vi "GitHub OAuth Test.vi"() -> ()   [LabVIEW 2013]
uses:
  source/OauthClient/OAuthClient.lvclass
  source/Oauth2/Oauth2.lvclass/Oauth2.ctl
  source/Oauth2/Oauth2.lvclass
  source/Oauth2.Github/Oauth2.GitHub.lvclass
  <vilib>/LabVIEW Open Source Project/OpenURI/uri/URI.lvclass
  <vilib>/httpClient/LabVIEWHTTPClient.lvlib
panel:
  out "GitHub Root":string
  out "HTTP Response Headers":string
  in  "login":string
  out "error out":errorcluster
  out "GitHub Access Token":string
  in  "GitHub Client Secret":string
  in  "GitHub Client ID":string
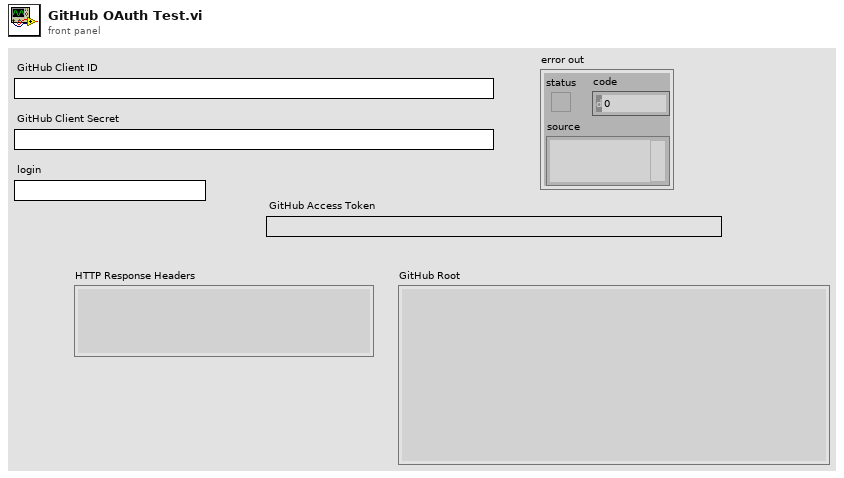
[diagram p1: front panel]
types:
  T1 = typedef "LabVIEWHTTPClient.lvlib/ClientHandle.ctl" = refnum<k1>
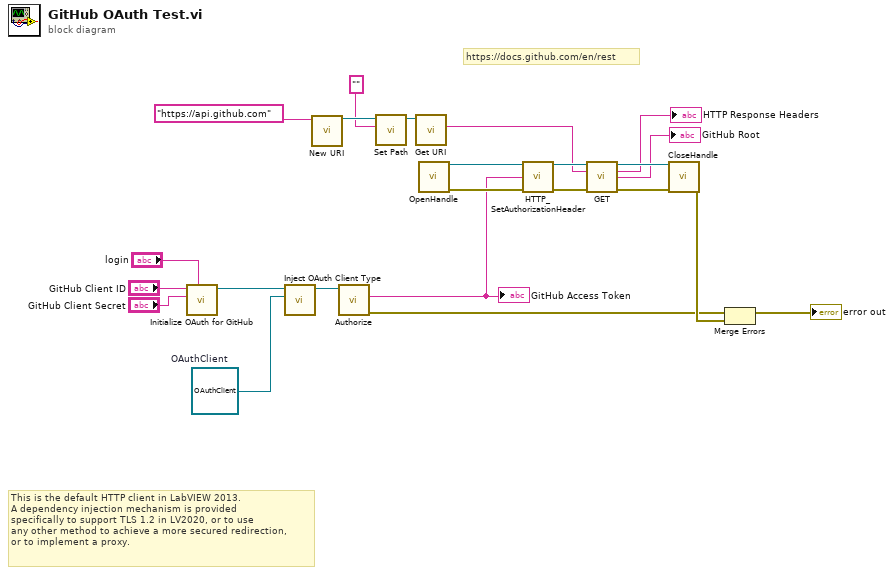
[diagram p0: block diagram]
diagram:
  w22 = refnum<class "OAuthClient.lvclass"> refnum  # OAuthClient
  # "https://docs.github.com/en/rest"
  # "This is the default HTTP client in LabVIEW 2013.\nA dependency injection mechanism is provided\nspecifically to support TLS 1.2 in LV2020, or to use\nany other method to achieve a more secured redirection, \nor to implement a proxy."
  n1 = call "Initialize OAuth for GitHub.vi"("login"="login", "Client Secret"="GitHub Client Secret", "Client ID"="GitHub Client ID") -> ("Oauth2.GitHub"=w19:refnum<class "Oauth2.GitHub.lvclass">)  [unwired: 8 in]
  n2 = call "Inject OAuth Client Type.vi"("OAuthClient"=w22, "Oauth2 in"=w19) -> ("Oauth2 out"=w23:refnum<class "Oauth2.GitHub.lvclass">)  [unwired: 9 in]
  n3 = call <vilib>:"New URI.vi"("URI"="https://api.github.com" ("path")) -> ("URI"=w17:refnum<class "URI.lvclass">)  [unwired: 9 in, 1 out]
  n4 = call "Authorize.vi"("Oauth2 in"=w23) -> ("error out"=w2:errorcluster, "Access Token"=w3:string)  [unwired: 8 in, 1 out]
  "GitHub Access Token" <- w3
  n5 = call <vilib>:"Set Path.vi"("path"="", "URI in"=w17) -> ("URI out"=w15:refnum<class "URI.lvclass">)  [unwired: 8 in, 1 out]
  n6 = call <vilib>:"Get URI.vi"("URI in"=w15) -> ("URI String"=w8:string)  [unwired: 8 in, 2 out]
  n7 = call <vilib>:"OpenHandle.vi"() -> ("client handle out"=w14:T1, "error out"=w13:errorcluster)  [unwired: 14 in]
  n8 = call "HTTP_SetAuthorizationHeader.vi"("Client Handle"=w14, "Access Token"=w3, "error in (no error)"=w13) -> ("client handle dup"=w12:T1, "error out"=w11:errorcluster)  [unwired: 11 in]
  n9 = call <vilib>:"GET.vi"("client handle"=w12, "url"=w8, "error in (no error)"=w11) -> ("client handle out"=w10:T1, "headers"=→"HTTP Response Headers":string, "body"=→"GitHub Root":string, "error out"=w9:errorcluster)  [unwired: 9 in]
  n10 = call <vilib>:"CloseHandle.vi"("client handle"=w10, "error in (no error)"=w9) -> ("error out"=w5:errorcluster)  [unwired: 13 in]
  n11 = Merge Errors(w2, w5) -> (→"error out":errorcluster)
